vi "Begin.vi"(8 "error in":errorcluster) -> (0 "error out":errorcluster)   [LabVIEW 2020]
doc: "Called before other user functions, this VI can be used to open I/O refnums, load in file data, and do general program initialization. Notice that the <B>error out</B> terminal is simply used for data flow. Wiring it to other structures or subVIs ensures that this VI runs first."
uses:
  <vilib>/Rock Robotics/WPI/DriverStation/WPI_DriverStationRobotMode2.ctl
  <vilib>/Rock Robotics/WPI/Joystick/WPI_JoystickDeviceEnum.ctl
  Robot Global Data.vi
  <vilib>/Rock Robotics/Network Tables/NT Write String Array.vi
  <vilib>/Rock Robotics/Network Tables/NT Read Boolean.vi
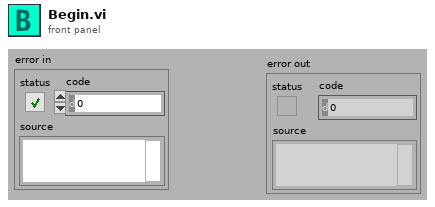
[diagram p1: front panel]
types:
  T1 = cluster{"Field Centric?":bool, "SnapToScore":bool, "TranslationalAlign":bool}
  T2 = typedef "WPI_JoystickDeviceEnum.ctl" = enum16{"USB 0", "USB 1", "USB 2", "USB 3", "USB 4", "USB 5"}
  T3 = typedef "WPI_DriverStationRobotMode2.ctl" = enum16{"Autonomous Disabled", "Autonomous Enabled", "Teleop Disabled", "Teleop Enabled", "Disconnected", "Finish", "Test Disabled", "Test Enabled", "Emergency Stopped"}
  T4 = typedef "WPI_JoystickDevRef.ctl" = cluster{"Device":T2}
  T5 = typedef "CTRE_PigeonIMU_DeviceRef.ctl" = cluster{"DeviceStatus":errorcluster, "Device Number":u8, "Type":T6, "Device ID":u32, "Handle":u64, "UsageFrame":u32, "Library Path":path}
  T6 = typedef "CTRE_PigeonIMU_ConnectionType.ctl" = u32
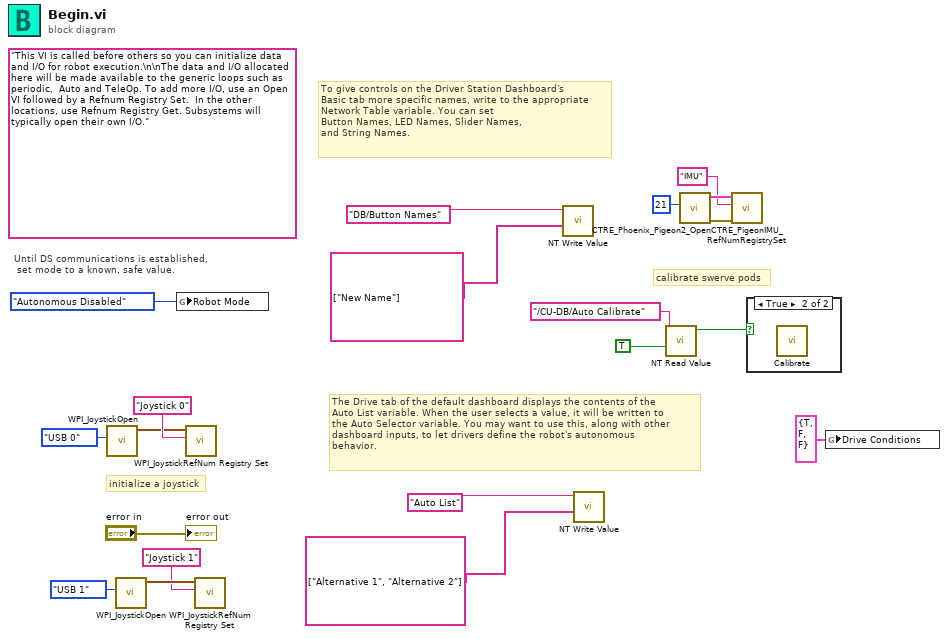
[diagram p0: block diagram]
diagram:
  (unwired) "This VI is called before others so you can initialize data and I/O for robot execution.\n\nThe data and I/O allocated here will be made available to the generic loops such as periodic,  Auto and TeleOp. To add more I/O, use an Open VI followed by a Refnum Registry Set.  In the other locations, use Refnum Registry Get. Subsystems will typically open their own I/O."
  # "calibrate swerve pods"
  # "The Drive tab of the default dashboard displays the contents of the\nAuto List variable. When the user selects a value, it will be written to\nthe Auto Selector variable. You may want to use this, along with other\ndashboard inputs, to let drivers define the robot's autonomous\nbehavior."
  # "To give controls on the Driver Station Dashboard's\nBasic tab more specific names, write to the appropriate\nNetwork Table variable. You can set\nButton Names, LED Names, Slider Names,\nand String Names."
  # "initialize a joystick"
  # "Until DS communications is established,\n set mode to a known, safe value."
  n1 = call <vilib>:"WPI_JoystickOpen.vi"("JoystickDevice"=WPI_JoystickDeviceEnum."USB 0") -> ("JoystickDevRef"=w18:T4)  [unwired: 10 in]
  n2 = call <vilib>:"WPI_JoystickOpen.vi"("JoystickDevice"=WPI_JoystickDeviceEnum."USB 1") -> ("JoystickDevRef"=w6:T4)  [unwired: 10 in]
  n3 = global write "Robot Global Data.vi" "Robot Mode"(WPI_DriverStationRobotMode2."Autonomous Disabled" ("Robot Mode")) -> ()
  n4 = call <vilib>:"WPI_JoystickRefNum Registry Set.vi"("refnum name"="Joystick 0", "JoystickDevRef"=w18) -> ()  [unwired: 8 in, 2 out]
  n5 = call <vilib>:"WPI_JoystickRefNum Registry Set.vi"("refnum name"="Joystick 1", "JoystickDevRef"=w6) -> ()  [unwired: 8 in, 2 out]
  n6 = call-poly <vilib>:"NT Write Value.vi"("value"=string[] ["New Name"] ("String Array"), "name"="DB/Button Names" ("Name")) -> ()  [unwired: 9 in, 1 out]
  n7 = call-poly <vilib>:"NT Write Value.vi"("value"=string[] ["Alternative 1", "Alternative 2"] ("String Array"), "name"="Auto List" ("Name")) -> ()  [unwired: 9 in, 1 out]
  n8 = call-poly <vilib>:"NT Read Value.vi"("default value"=TRUE, "name"="/CU-DB/Auto Calibrate") -> ("value"=w2:bool)  [unwired: 7 in, 2 out]
  n9 = call <vilib>:"CTRE_Phoenix_Pigeon2_Open.vi"("Device Number"=u8 21) -> ("error out"=w11:errorcluster, "PigeonIMUDevRef"=w10:T5)  [unwired: 9 in]
  n10 = call <vilib>:"CTRE_PigeonIMU_RefNumRegistrySet.vi"("error in (no error)"=w11, "refnum name"="IMU", "PigeonIMUDevRef"=w10) -> ()  [unwired: 7 in, 2 out]
  n11 = case shown="True" w2 {
    frame False {
    }
    frame True {
      n12 = call "Calibrate.vi"() -> ()  [unwired: 11 in, 1 out]
    }
  }
  n13 = global write "Robot Global Data.vi" "Drive Conditions"(T1 {"Field Centric?"=TRUE, "SnapToScore"=FALSE, "TranslationalAlign"=FALSE} ("Drive Conditions")) -> ()
  "error out" <- "error in"
